vi "goal_circle_constraint.vi"(9 "Goal tip pos":sgl[](array[numeric]), 10 "Goal pose (handle basis) in":T12, 11 "Parameters":T1={"Stimulus"={"Type"=enum."Off", "Phase"=0.0, "Amplitude"=[], "Injection point"=enum."Total pose", "Closed loop"=FALSE, "Offset"=[], "Tip -> world"=FALSE, "Frequency"=0.0, "Length"=0.0}, "Goal Filter A"={"Speedup max"=0.0, "Speedup thresh"=0.0, "Speedup nonlin"=0.0, "Filters"=[]}, "Mode controls"={"Hold"=FALSE, "Cancellation"=FALSE, "Goal filter"=FALSE, "Trigger"=FALSE}, "Manipulator type"=enum."Current piezo", "Manipulator calibration"={"Tool offsets"=[[0.0, 0.0, 36200.0]], "Handle light calibration"=[], "Base pivots"=[], "Output pivots"=[], "Length center"=0.0, "Workspace height"=[], "Workspace diameter"=[0.0, 0.0, 36200.0], "Stack travel"=400.0, "Saturation pos"=375.0, "Inverse filters"=[], "Strut length"=0.0}, "Network"={"Remote Host"="", "Send Status"=FALSE, "Send Port"=0, "Recv Commands"=FALSE, "Recv Port"=0}, "Goal Filter B"={"Speedup max"=0.0, "Speedup thresh"=0.0, "Speedup nonlin"=0.0, "Filters"=[]}, "Cancellation"={"KP"={"XY"=0.0, "Rxy"=0.0, "Z"=0.0, "Rz"=0.0}, "KI"=0.0, "KD"={"XY"=0.0, "Rxy"=0.0, "Z"=0.0, "Rz"=0.0}, "Max vel"=20.0, "Max acc"=0.001, "Int error limit"=3.0, "RCM gain"=0.0, "Bypass"=FALSE, "Degraded gain"=0.0}, "Transition time"=0.0, "Estimation"={"Link"={"Measure noise"=[], "Process noise"=[], "Alt process noise"=[], "Alt turnoff cycles"=20, "Innovation limit"=[], "Residue threshold"=0.0, "Enable"=FALSE}, "Handle"={"Measure noise"=[], "Process noise"=[], "State limits"=[], "Innovation limit"=[], "Prediction Lookahead"=0.0, "Enable"=FALSE}}} {"Transition time" format="%_3f"; "Cancellation"."Degraded gain" min=0 max=1 step=0.1 format="%#_3p"; "Cancellation"."RCM gain" min=0 max=1 step=0.1 format="%#_3p"; "Cancellation"."KD"."Rz" min=-1 max=1 step=0.01 format="%#_3p"; "Cancellation"."KD"."Rxy" min=-1 max=1 step=0.01 format="%#_3p"; "Cancellation"."KD"."Z" min=-1 max=1 step=0.01 format="%#_3p"; "Cancellation"."KD"."XY" min=-1 max=1 step=0.01 format="%#_3p"; "Cancellation"."KI" min=0 max=1 step=0.01 format="%#_3p"; "Cancellation"."KP"."Rz" min=-1 max=1 step=0.01 format="%#_3p"; "Cancellation"."KP"."Rxy" min=-1 max=1 step=0.01 format="%#_3p"; "Cancellation"."KP"."Z" min=-1 max=1 step=0.01 format="%#_3p"; "Cancellation"."KP"."XY" min=-1 max=1 step=0.01 format="%#_3p"; "Cancellation"."Max acc" format="%#_3p"; "Goal Filter B"."Filters"."V limit range" format="%_3p"; "Goal Filter B"."Filters"."V limit" format="%_3p"; "Goal Filter B"."Filters"."Upper Q" format="%_3f"; "Goal Filter B"."Filters"."Upper Fc" format="%_3p"; "Goal Filter B"."Filters"."Lower Q" format="%_3f"; "Goal Filter B"."Filters"."Scale factor" format="%_3f"; "Goal Filter B"."Filters"."Lower Fc" format="%_3p"; "Goal Filter B"."Speedup nonlin" format="%_3p"; "Goal Filter B"."Speedup thresh" format="%_3p"; "Goal Filter B"."Speedup max" format="%_3p"; "Manipulator calibration"."Strut length" format="%#_4p"; "Manipulator calibration"."Saturation pos" format="%#.1f"; "Manipulator calibration"."Stack travel" format="%#.1f"; "Manipulator calibration"."Length center" format="%#_4p"; "Manipulator calibration"."Output pivots" format="%#_6f"; "Manipulator calibration"."Base pivots" format="%#_6f"; "Manipulator calibration"."Handle light calibration" format="%#.1f"; "Goal Filter A"."Filters"."V limit range" format="%_3p"; "Goal Filter A"."Filters"."V limit" format="%_3p"; "Goal Filter A"."Filters"."Upper Q" format="%_3f"; "Goal Filter A"."Filters"."Upper Fc" format="%_3p"; "Goal Filter A"."Filters"."Lower Q" format="%_3f"; "Goal Filter A"."Filters"."Scale factor" format="%_3f"; "Goal Filter A"."Filters"."Lower Fc" format="%_3p"; "Goal Filter A"."Speedup nonlin" format="%_3p"; "Goal Filter A"."Speedup thresh" format="%_3p"; "Goal Filter A"."Speedup max" format="%_3p"; "Stimulus"."Length" min=0.0 max=100.0 step=100.0 format="%#_4p"; "Stimulus"."Frequency" min=0.0 step=100.0 format="%#_4g"; "Stimulus"."Offset" format="%#_3p"; "Stimulus"."Amplitude" format="%#_3p"; "Stimulus"."Phase" min=-180.0 max=360.0 step=100.0 format="%#.2f"}) -> (0 "Saturation":bool, 3 "Goal pose (handle basis) out":T12, 4 "Clip point":sgl[][](array[numeric]))   [LabVIEW 2014]
uses:
  <vilib>/Analysis/Matrix/Datatypes/RealMatrix.ctl
  testing/Micron params.ctl
  testing/stimulus.ctl
  testing/injection_point.ctl
  goal_loop_parms.ctl
  testing/mode_conrols.ctl
  testing/manipulator_cal.ctl
  asap/labview/testing/probe_calibration.ctl
  host/network_params.ctl
  cancellation/sq_control_params.ctl
  cancellation/decoupled_gain.ctl
  cancellation/estimation_controls.ctl
  utilities/labview/norm_vec_single.vi
  <vilib>/Analysis/Matrix/NI_Matrix.lvlib
panel:
  # "Limit goal pose to meet circle constraint.  If \"Saturation\" is false, then the output is identical to the input pose."
  # "If saturated, this is the nominal and goal position of the limit circle point after clipping to fit the workspace."
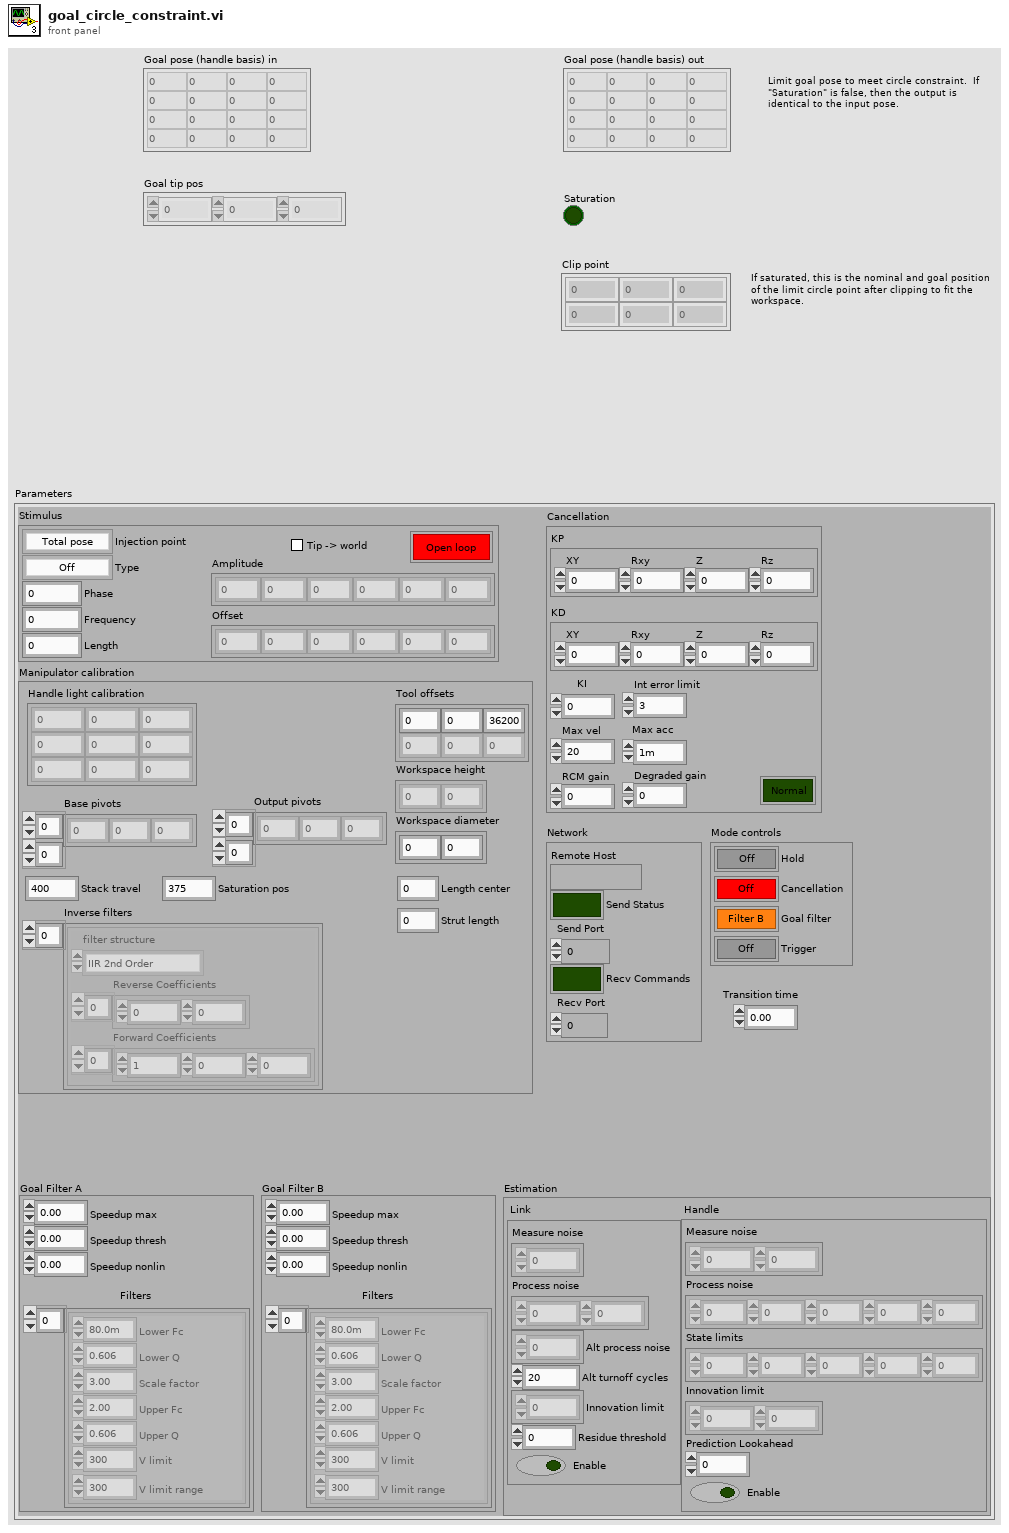
[diagram p1: front panel]
types:
  T1 = typedef "Micron params.ctl" = cluster{"Stimulus":T2, "Goal Filter A":T4, "Mode controls":T5, "Manipulator type":enum16{"Current piezo", "Voltage piezo"}, "Manipulator calibration":T6, "Network":T8, "Goal Filter B":T4, "Cancellation":T9, "Transition time":sgl, "Estimation":T11}
  T2 = typedef "stimulus.ctl" = cluster{"Type":enum16{"Off", "Step", "Sine", "Triangle", "Arbitrary"}, "Phase":dbl, "Amplitude":sgl[], "Injection point":T3, "Closed loop":bool, "Offset":sgl[], "Tip -> world":bool, "Frequency":dbl, "Length":dbl}
  T3 = typedef "injection_point.ctl" = enum16{"Total pose", "V limiter", "Goal ", "Link position", "KF link position", "Inverse kin", "Link goal", "Link error", "Controller", "Output", "Drive", "Light"}
  T4 = typedef "goal_loop_parms.ctl" = cluster{"Speedup max":sgl, "Speedup thresh":sgl, "Speedup nonlin":sgl, "Filters":cluster{"Lower Fc":sgl, "Lower Q":sgl, "Scale factor":sgl, "Upper Fc":sgl, "Upper Q":sgl, "V limit":sgl, "V limit range":sgl}[]}
  T5 = typedef "mode_conrols.ctl" = cluster{"Hold":bool, "Cancellation":bool, "Goal filter":bool, "Trigger":bool}
  T6 = typedef "manipulator_cal.ctl" = cluster{"Tool offsets":sgl[][], "Handle light calibration":T7, "Base pivots":sgl[][], "Output pivots":sgl[][], "Length center":sgl, "Workspace height":sgl[], "Workspace diameter":sgl[], "Stack travel":sgl, "Saturation pos":sgl, "Inverse filters":cluster{"filter structure":enum32{"IIR 2nd Order", "IIR 4th Order"}, "Reverse Coefficients":dbl[], "Forward Coefficients":dbl[]}[], "Strut length":sgl}
  T7 = typedef "probe_calibration.ctl" = sgl[][]
  T8 = typedef "network_params.ctl" = cluster{"Remote Host":string, "Send Status":bool, "Send Port":u16, "Recv Commands":bool, "Recv Port":u16}
  T9 = typedef "sq_control_params.ctl" = cluster{"KP":T10, "KI":sgl, "KD":T10, "Max vel":sgl, "Max acc":sgl, "Int error limit":sgl, "RCM gain":sgl, "Bypass":bool, "Degraded gain":sgl}
  T10 = typedef "decoupled_gain.ctl" = cluster{"XY":sgl, "Rxy":sgl, "Z":sgl, "Rz":sgl}
  T11 = typedef "estimation_controls.ctl" = cluster{"Link":cluster{"Measure noise":dbl[], "Process noise":dbl[], "Alt process noise":dbl[], "Alt turnoff cycles":i32, "Innovation limit":dbl[], "Residue threshold":dbl, "Enable":bool}, "Handle":cluster{"Measure noise":dbl[], "Process noise":dbl[], "State limits":dbl[], "Innovation limit":dbl[], "Prediction Lookahead":sgl, "Enable":bool}}
  T12 = typedef "NI_Matrix.lvlib/RealMatrix.ctl" = dbl[][]
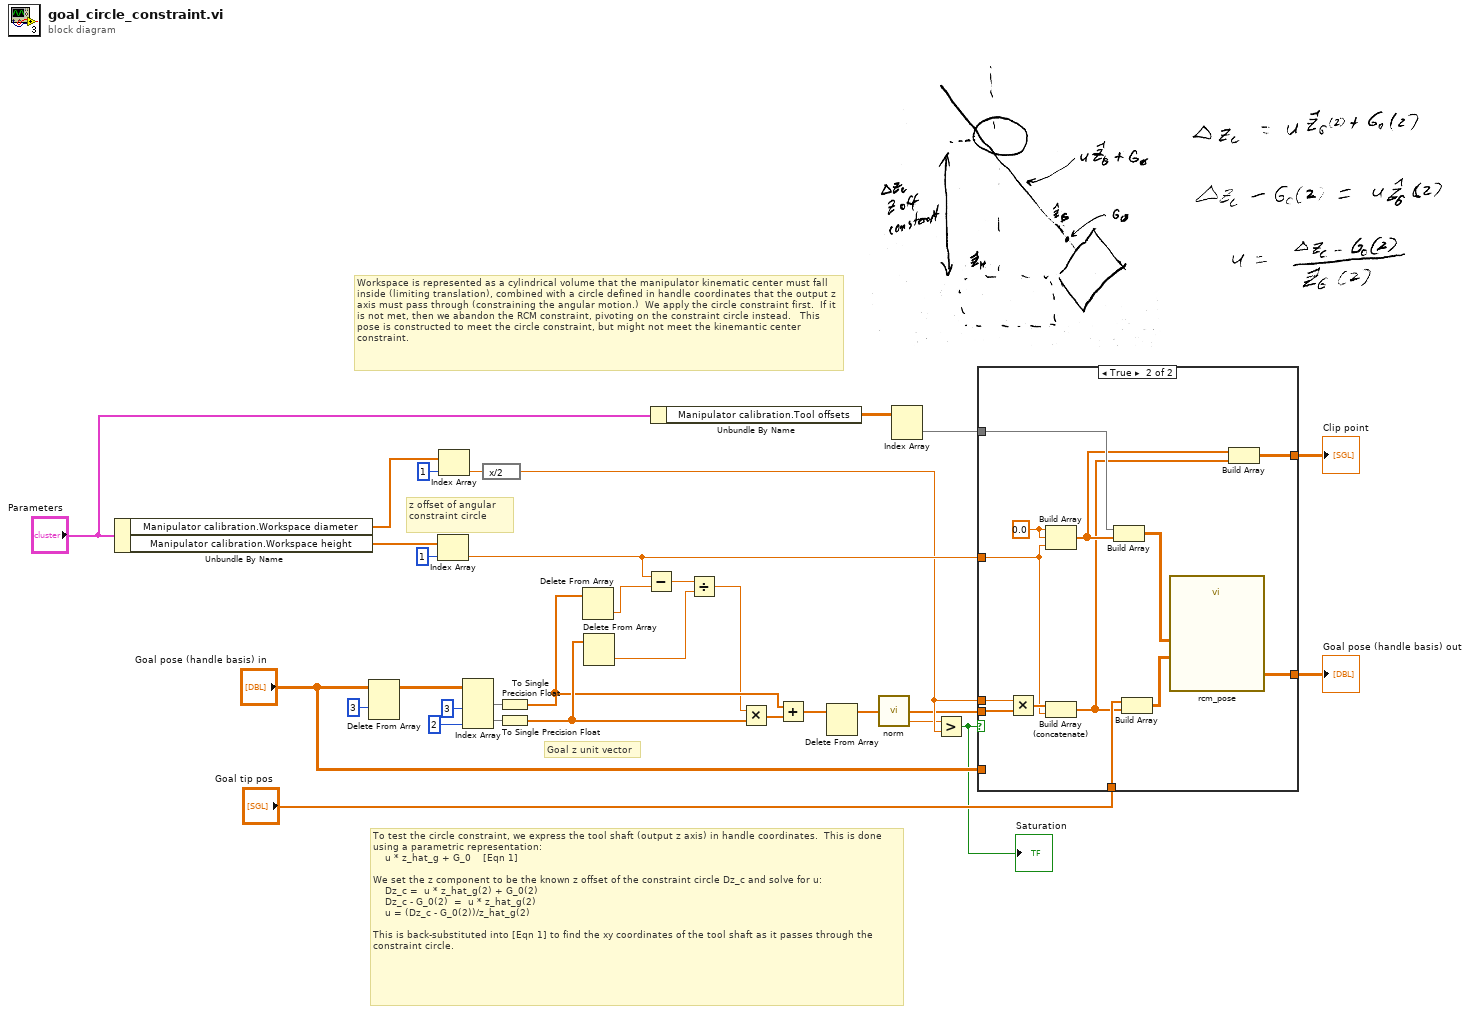
[diagram p0: block diagram]
diagram:
  # "To test the circle constraint, we express the tool shaft (output z axis) in handle coordinates.  This is done using a parametric representation:\n    u * z_hat_g + G_0    [Eqn 1]\n\nWe set the z component to be the known z offset of the constraint circle Dz_c and solve for u:\n    Dz_c =  u * z_hat_g(2) + G_0(2)\n    Dz_c - G_0(2)  =  u * z_hat_g(2) \n    u = (Dz_c - G_0(2))/z_hat_g(2)\n\nThis is back-substituted into [Eqn 1] to find the xy coordinates of the tool shaft as it passes through the constraint circle."
  # "Workspace is represented as a cylindrical volume that the manipulator kinematic center must fall inside (limiting translation), combined with a circle defined in handle coordinates that the output z axis must pass through (constraining the angular motion.)  We apply the circle constraint first.  If it is not met, then we abandon the RCM constraint, pivoting on the constraint circle instead.   This pose is constructed to meet the circle constraint, but might not meet the kinemantic center constraint."
  # "Goal z unit vector"
  # "z offset of angular constraint circle"
  n1 = Unbundle By Name("Parameters") -> ("Manipulator calibration.Workspace diameter"=w19:sgl[], "Manipulator calibration.Workspace height"=w2:sgl[])
  n2 = Delete From Array(array="Goal pose (handle basis) in", index (row)=3) -> (array with subset deleted=w5:T12)  [unwired: 2 in, 1 out]
  n3 = Index Array(array=w2, index=1) -> (element=w26:sgl)
  n4 = Index Array(array=w19, index=1) -> (element=w20:sgl)
  n5 = Index Array(array=w5, index (col) #1=3 ("disabled index (col)"), index (col) #2=2 ("index (col)")) -> (element #1=w13:dbl[], element #2=w15:dbl[])  [unwired: 2 in]
  n6 = expression code="x/2"(w20) -> (w25:sgl)
  n7 = To Single Precision Float(number=w13) -> (single precision float=w14:sgl[])
  n8 = To Single Precision Float(number=w15) -> (single precision float=w16:sgl[])
  n9 = Delete From Array(array=w14) -> (deleted portion=w8:sgl)  [unwired: 2 in, 1 out]
  n10 = Delete From Array(array=w16) -> (deleted portion=w10:sgl)  [unwired: 2 in, 1 out]
  n11 = Subtract(x=w26, y=w8) -> (x-y=w9:sgl)
  n12 = Unbundle By Name("Parameters") -> ("Manipulator calibration.Tool offsets"=w27:sgl[][])
  n13 = Divide(x=w9, y=w10) -> (x/y=w11:sgl)
  n14 = Multiply(x=w11, y=w16) -> (x*y=w12:sgl[])
  n15 = Add(x=w14, y=w12) -> (x+y=w17:sgl[])
  n16 = Delete From Array(array=w17) -> (array with subset deleted=w22:sgl[])  [unwired: 2 in, 1 out]
  n17 = call-poly "norm.vi"("vector"=w22) -> ("magnitude"=w23:sgl, "normalized vector"=w24:sgl[])  [unwired: 3 in]
  n18 = Index Array(array=w27) -> (element=w28:sgl[])  [unwired: 2 in]
  n19 = Greater?(x=w23, y=w25) -> (0:w21:bool)
  "Saturation" <- w21
  n20 = case shown="True" w21 {
    tunnel: w24 -> [_ w46]
    tunnel: w25 -> [_ w45]
    tunnel: w26 -> [_ w42]
    tunnel: w28 -> [_ w43]
    tunnel: "Goal tip pos" -> [_ w39]
    tunnel: [w33 w37] -> w31
    tunnel: "Goal pose (handle basis) in" -> [w33 _]
    tunnel: [_ w34] -> w1
    frame False {
    }
    frame True {
      w41 = sgl 0.0 ("Numeric")
      n21 = Multiply ("Multiply.vi")(x=w45, y=w46) -> (x*y=w44:sgl[])
      n22 = Build Array(w41, w41, w42) -> (w36:sgl[])
      n23 = Build Array (concatenate)(w44, w42) -> (w35:sgl[])
      n24 = Build Array(w43, w36) -> (w40:sgl[][])
      n25 = Build Array(w39, w35) -> (w38:sgl[][])
      n26 = call "rcm_pose.vi"("Goal positions"=w38, "Nominal positions"=w40) -> ("Goal pose (handle basis)"=w37:T12)  [unwired: 9 in]
      n27 = Build Array(w36, w35) -> (w34:sgl[][])
    }
  }
  "Goal pose (handle basis) out" <- w31
  "Clip point" <- w1
